vi "Read ADC Sim.vi"(8 "error in (no error)":errorcluster, 9 "Canal":u8, 10 "Device":string, 11 "Simulated in":refnum<class "Simulated.lvclass">) -> (0 "error out":errorcluster, 1 "Expected response":string, 3 "Simulated out":refnum<class "Simulated.lvclass">)   [LabVIEW 2020, in "Simulated.lvclass"]
uses:
  Simulated.lvclass
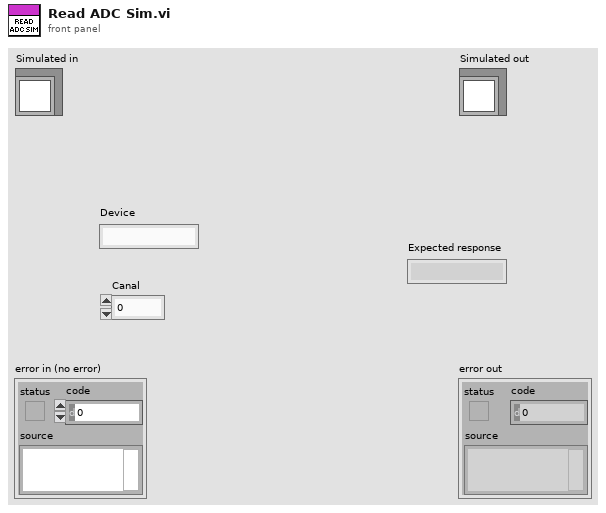
[diagram p1: front panel]
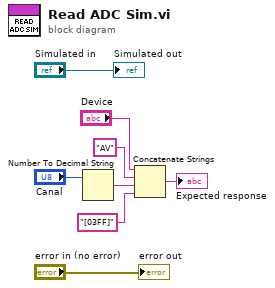
[diagram p0: block diagram]
diagram:
  n1 = Number To Decimal String(number="Canal") -> (decimal integer string=w3:string)  [unwired: 1 in]
  n2 = Concatenate Strings("Device", "AV" ("string"), w3, "[03FF]" ("string")) -> (→"Expected response":string)
  "error out" <- "error in (no error)"
  "Simulated out" <- "Simulated in"
